vi "get value for key.vi"(8 "error in":errorcluster, 10 "key":string, 11 "fixed channel configuration in":refnum<class "fixed channel configuration.lvclass">) -> (0 "error out":errorcluster, 1 "value":string, 3 "fixed channel configuration out":refnum<class "fixed channel configuration.lvclass">)   [LabVIEW 2013, in "fixed channel configuration.lvclass"]
uses:
  fixed channel configuration.lvclass
  fixed channel configuration.lvclass/fixed channel configuration.ctl
  <vilib>/NI/Configuration Framework/NISE_CEF_TreeControl.lvlib
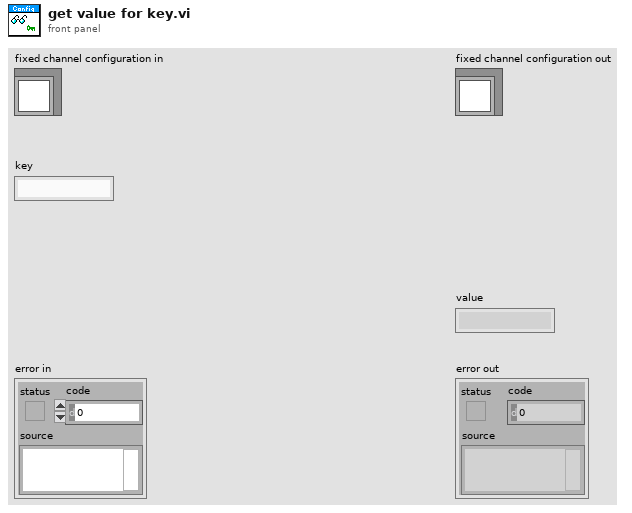
[diagram p1: front panel]
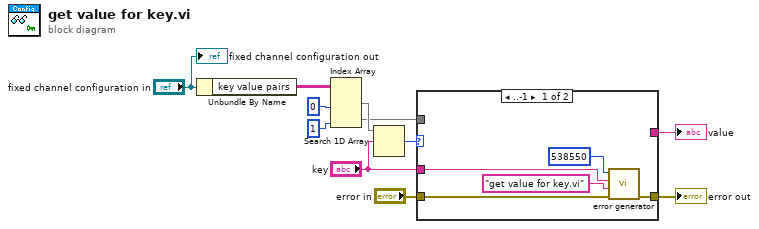
[diagram p0: block diagram]
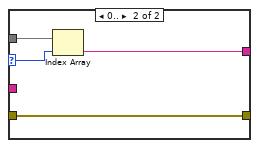
[diagram p2: hidden frame]
diagram:
  n1 = Unbundle By Name("fixed channel configuration in") -> ("key value pairs"=w10:string[][])
  n2 = Index Array(array=w10, index (col) #1=0 ("disabled index (col)"), index (col) #2=1 ("disabled index (col)")) -> (element #1=w7:string[], element #2=w5:string[])  [unwired: 2 in]
  n3 = Search 1D Array(1D array=w7, element="key") -> (index of element=w6:i32)  [unwired: 1 in]
  n4 = case shown="..-1" w6 {
    selector: w6 -> [_ w19]
    tunnel: w5 -> [_ w20]
    tunnel: [_ w18] -> w4
    tunnel: "error in" -> [w14 w17]
    tunnel: [w13 w17] -> w2
    tunnel: "key" -> [w12 _]
    frame ..-1 {
      n5 = call <vilib>:"error generator.vi"("error in"=w14, "source"="get value for key.vi", "append error message"=w12, "error code (0)"=538550) -> ("error out"=w13:errorcluster)  [unwired: 5 in]
    }
    frame 0.. {
      n6 = Index Array(array=w20, index=w19) -> (element=w18:string)
    }
  }
  "value" <- w4
  "error out" <- w2
  "fixed channel configuration out" <- "fixed channel configuration in"
